vi "build token URI.vi"(8 "error in (no error)":errorcluster, 11 "Oauth2 in":refnum<class "Oauth2.lvclass">) -> (0 "error out":errorcluster, 2 "Token Request URI":string, 3 "Oauth2":refnum<class "Oauth2.lvclass">)   [LabVIEW 2013, in "Oauth2.lvclass"]
uses:
  Oauth2.lvclass
  OAuthToken/OAuth2 Token Element -- enum.ctl
  Oauth2.lvclass/Oauth2.ctl
  <vilib>/LabVIEW Open Source Project/OpenURI/uri/URI.lvclass
  OAuthToken/OAuthAccessToken.lvclass
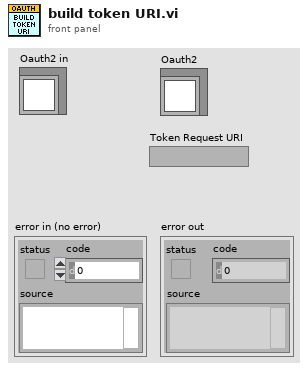
[diagram p1: front panel]
types:
  T1 = typedef "OAuthAccessToken.lvclass/OAuth2 Token Element -- enum.ctl" = enum16{"client_id", "client_secret", "response_type", "scope", "redirect_uri", "error", "error_description", "error_uri", "grant_type", "code", "access_token", "token_type", "expires_in", "username", "password", "refresh_token", "code_challenge", "code_challenge_method", "endpoint element"}
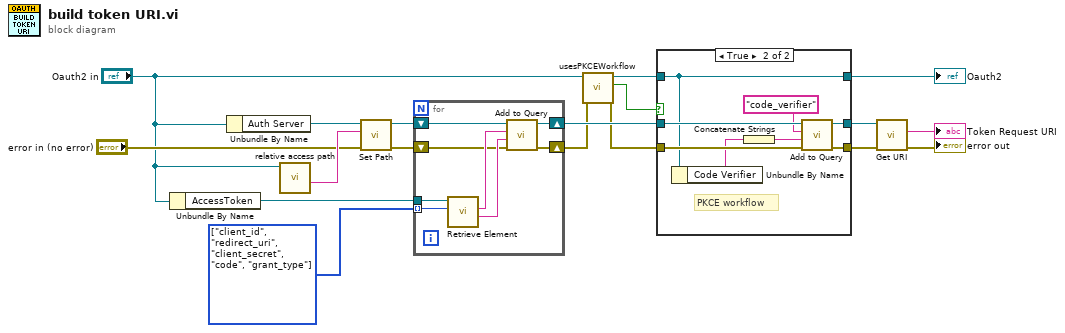
[diagram p0: block diagram]
diagram:
  w12 = T1[] [enum."client_id", enum."redirect_uri", enum."client_secret", enum."code", enum."grant_type"] items=["client_id", "client_secret", "response_type", "scope", "redirect_uri", "error", "error_description", "error_uri", "grant_type", "code", "access_token", "token_type", "expires_in", "username", "password", "refresh_token", "code_challenge", "code_challenge_method", "endpoint element"]
  n1 = Unbundle By Name("Oauth2 in") -> ("AccessToken"=w13:refnum<class "OAuthAccessToken.lvclass">)
  n2 = Unbundle By Name("Oauth2 in") -> ("Auth Server"=w15:refnum<class "URI.lvclass">)
  n3 = call-dynamic "relative access path.vi"("Oauth2 in"="Oauth2 in") -> ("Token Access Path"=w16:string)  [unwired: 9 in, 1 out]
  n4 = call <vilib>:"Set Path.vi"("error in (no error)"="error in (no error)", "path"=w16, "URI in"=w15) -> ("error out"=w10:errorcluster, "URI out"=w11:refnum<class "URI.lvclass">)  [unwired: 7 in]
  n5 = for {
    tunnel: w13 -> [w26]
    tunnel: w12 -> [w25] mode=indexing
    shift-right: [w23] -> w9
    shift-left: w11 -> [w24]
    shift-right: [w19] -> w5
    shift-left: w10 -> [w20]
    n6 = call "Retrieve Element.vi"("Token element"=w25, "OAuthAccessToken in"=w26) -> ("Value"=w21:string, "Key"=w22:string)  [unwired: 5 in, 3 out]
    n7 = call <vilib>:"Add to Query.vi"("error in (no error)"=w20, "value"=w21, "key"=w22, "URI in"=w24) -> ("error out"=w19:errorcluster, "URI out"=w23:refnum<class "URI.lvclass">)  [unwired: 6 in]
  }
  n8 = call "usesPKCEWorkflow.vi"("error in (no error)"=w5, "Oauth2 in"="Oauth2 in") -> ("error out"=w4:errorcluster, "PKCE?"=w3:bool, "Oauth2 out"=w2:refnum<class "Oauth2.lvclass">)  [unwired: 7 in]
  n9 = case shown="True" w3 {
    tunnel: w9 -> [w28 w37]
    tunnel: [w28 w36] -> w8
    tunnel: w4 -> [w29 w35]
    tunnel: [w29 w34] -> w7
    tunnel: w2 -> [w27 w32]
    tunnel: [w27 w32] -> w1
    frame False {
    }
    frame True {
      # "PKCE workflow"
      n10 = Unbundle By Name(w32) -> ("Code Verifier"=w31:string)
      n11 = Concatenate Strings(w31) -> (w30:string)
      n12 = call <vilib>:"Add to Query.vi"("error in (no error)"=w35, "value"=w30, "key"="code_verifier", "URI in"=w37) -> ("error out"=w34:errorcluster, "URI out"=w36:refnum<class "URI.lvclass">)  [unwired: 6 in]
    }
  }
  "Oauth2" <- w1
  n13 = call <vilib>:"Get URI.vi"("error in (no error)"=w7, "URI in"=w8) -> ("error out"=→"error out":errorcluster, "URI String"=→"Token Request URI":string)  [unwired: 7 in, 1 out]
